vi "GetToolbarButtons.vi"(0 "reference":refnum<class "Graph.lvclass">, 2 "GraphButton":u32, 5 "error in (no error)":errorcluster) -> (14 "reference out":refnum<class "Graph.lvclass">, 15 "AllToolbarButtons":T2[](array[typedef]), 16 "Text":string, 17 "Type":T1, 19 "error out":errorcluster)   [LabVIEW 2016, in "Graph.lvclass"]
doc: "public boolean add(Node n, Point2D p)"
uses:
  <resource>/Framework/Providers/Open_GDS/UML/Graph_class/Graph.lvclass
  <resource>/Framework/Providers/Open_GDS/UML/Graph_class/ToolbarButtonType.ctl
  <resource>/Framework/Providers/Open_GDS/UML/UMLEditor/UMLEditor tooltype.ctl
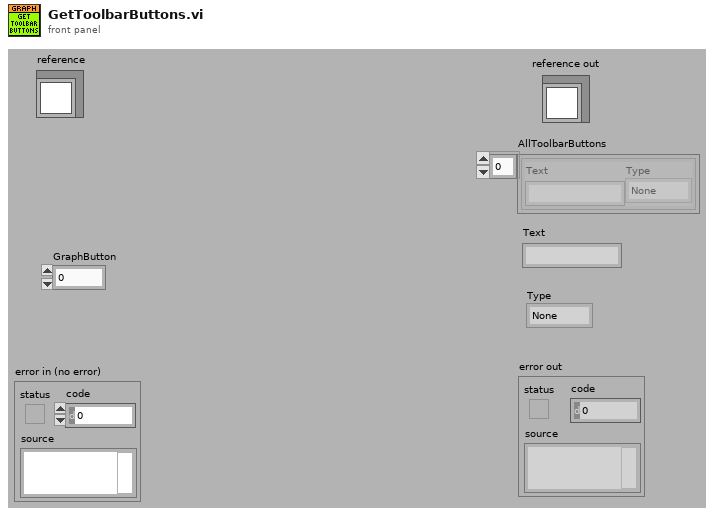
[diagram p1: front panel]
types:
  T1 = typedef "UMLEditor tooltype.ctl" = enum16{"None", "Node", "Edge"}
  T2 = typedef "Graph.lvclass/ToolbarButtonType.ctl" = cluster{"Text":string, "Type":T1}
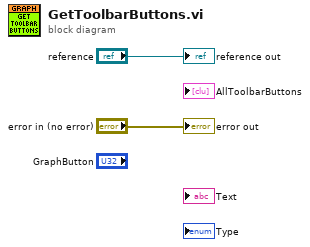
[diagram p0: block diagram]
diagram:
  "reference out" <- "reference"
  "error out" <- "error in (no error)"
